vi "Problem 19.vi"() -> ()   [LabVIEW 2013, in "Problem 19.lvlib"]
uses:
  Problem 19.lvlib
panel:
  out "# Sundays":i32
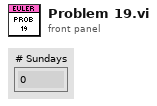
[diagram p1: front panel]
types:
  T1 = typedef "LVDateTimeRec.ctl" = cluster{"fractional second":dbl, "second":i32, "minute":i32, "hour":i32, "day of month":i32, "month":i32, "year":i32, "day of week":i32, "day of year":i32, "DST":i32}
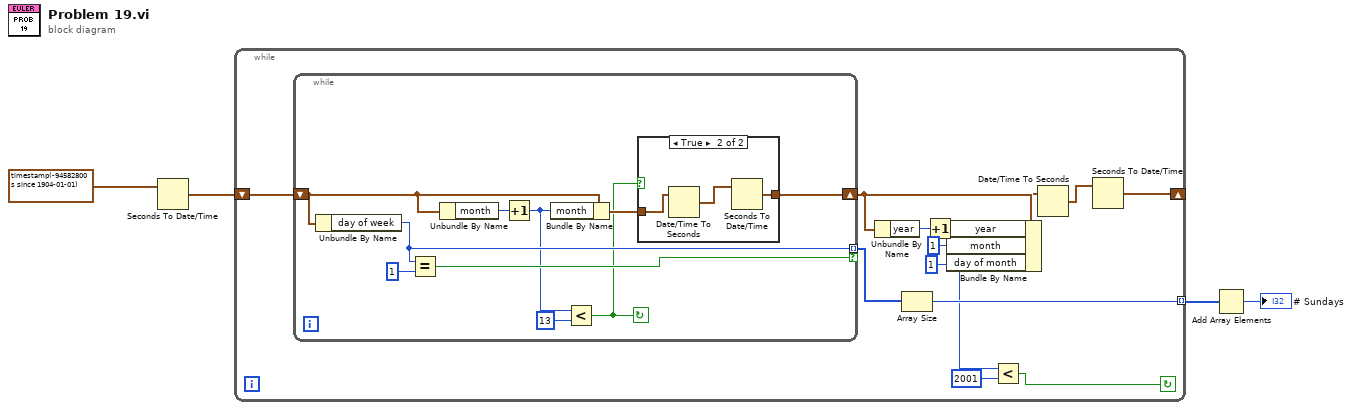
[diagram p0: block diagram]
diagram:
  n1 = Seconds To Date/Time(time stamp (now)=timestamp(-94582800 s since 1904-01-01)) -> (date time rec=w3:T1)  [unwired: 1 in]
  n2 = while {
    shift-right: [w11] -> _
    shift-left: w3 -> [w17]
    tunnel: [w9] -> w2 mode=indexing
    stop <- w6 continue-if-true
    n3 = while {
      tunnel: [w26] -> w10 mode=indexing if=w25
      shift-right: [w20] -> w16
      shift-left: w17 -> [w21]
      stop <- w18 continue-if-true
      n4 = Unbundle By Name(w21) -> ("day of week"=w26:i32)
      n5 = Equal?(x=w26, y=1) -> (x = y?=w25:bool)
      n6 = Unbundle By Name(w21) -> ("month"=w24:i32)
      n7 = Increment(x=w24) -> (x+1=w23:i32)
      n8 = Bundle By Name(cluster=w21, "month"=w23) -> (w19:T1)
      n9 = Less?(x=w23, y=13) -> (x < y?=w18:bool)
      n10 = case shown="True" w18 {
        tunnel: [w28 w30] -> w20
        tunnel: w19 -> [w28 w29]
        frame False {
        }
        frame True {
          n11 = Date/Time To Seconds(2:w29) -> (0:w31:timestamp)  [unwired: 1 in]
          n12 = Seconds To Date/Time(time stamp (now)=w31) -> (date time rec=w30:T1)  [unwired: 1 in]
        }
      }
    }
    n13 = Unbundle By Name(w16) -> ("year"=w15:i32)
    n14 = Array Size(array=w10) -> (size(s)=w9:i32)
    n15 = Increment(x=w15) -> (x+1=w8:i32)
    n16 = Bundle By Name(cluster=w16, "year"=w8, "month"=1, "day of month"=1) -> (w12:T1)
    n17 = Less?(x=w8, y=2001) -> (x < y?=w6:bool)
    n18 = Date/Time To Seconds(2:w12) -> (0:w13:timestamp)  [unwired: 1 in]
    n19 = Seconds To Date/Time(time stamp (now)=w13) -> (date time rec=w11:T1)  [unwired: 1 in]
  }
  n20 = Add Array Elements(numeric array=w2) -> (sum=→"# Sundays":i32)
